vi "Vision Test.vi"() -> ()   [LabVIEW 2011]
panel:
  out "Number of Targets":i32(slide) scale=0.005..5.0
  in  "Margin of Error":i32=25
  in  "Draw Targets":bool
  out "Procesing Time":cluster{"Procesing Time":u32, "CAi":dbl}(graph)
  in  "stop":bool
  in  "Blue or Luma or Val or Inten Range":cluster{"Lower value":i32, "Upper value":i32}={"Lower value"=20, "Upper value"=120}
  in  "Green or Sat Range":cluster{"Lower value":i32, "Upper value":i32}={"Lower value"=0, "Upper value"=255}
  in  "Red or Hue Range":cluster{"Lower value":i32, "Upper value":i32}={"Lower value"=80, "Upper value"=100}
  out "ImageR":T1(plugin-control)
  out "ImageL":T1(plugin-control)
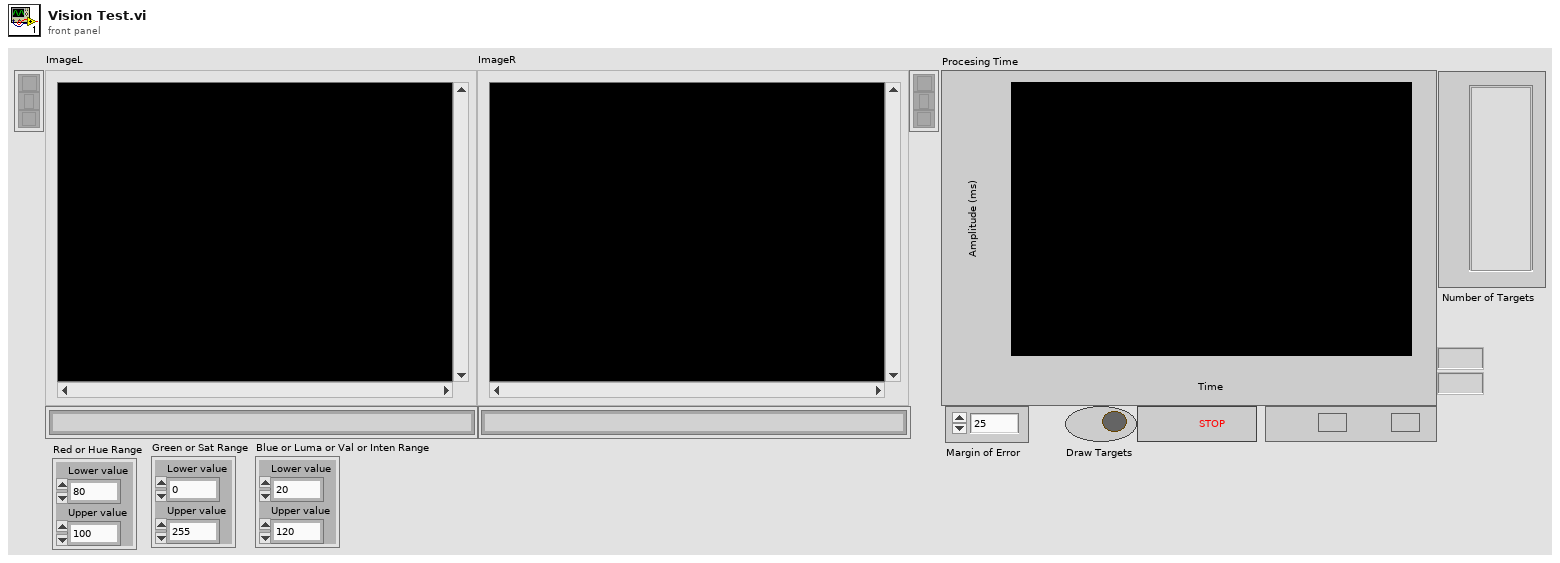
[diagram p1: front panel]
types:
  T1 = typedef "IMAQ Image.ctl" = refnum<image>
  T2 = typedef "Image Type" = u32
  T3 = cluster{"LeftImage_Mark":cluster{"Blob":cluster{"Center of Mass":cluster{"X":dbl, "Y":dbl}, "First Pixel":cluster{"X":dbl, "Y":dbl}, "Bounding Rect":cluster{"Left":dbl, "Top":dbl, "Right":dbl, "Bottom":dbl}, "Bounding Rect Size":cluster{"X":dbl, "Y":dbl}, "Area":dbl}, "Cluster":cluster{"TopLeft":cluster{"X":dbl, "Y":dbl}, "TopRight":cluster{"X":dbl, "Y":dbl}, "BottomRight":cluster{"X":dbl, "Y":dbl}, "BottomLeft":cluster{"X":dbl, "Y":dbl}}}, "RightImage_Mark":cluster{"Blob":cluster{"Center of Mass":cluster{"X":dbl, "Y":dbl}, "First Pixel":cluster{"X":dbl, "Y":dbl}, "Bounding Rect":cluster{"Left":dbl, "Top":dbl, "Right":dbl, "Bottom":dbl}, "Bounding Rect Size":cluster{"X":dbl, "Y":dbl}, "Area":dbl}, "Cluster":cluster{"TopLeft":cluster{"X":dbl, "Y":dbl}, "BottomRight":cluster{"X":dbl, "Y":dbl}, "BottomLeft":cluster{"X":dbl, "Y":dbl}, "TopRight":cluster{"X":dbl, "Y":dbl}}}, "Numeric Control":dbl}[]
  T4 = cluster{"Procesing Time":u32, "Running Average":dbl}
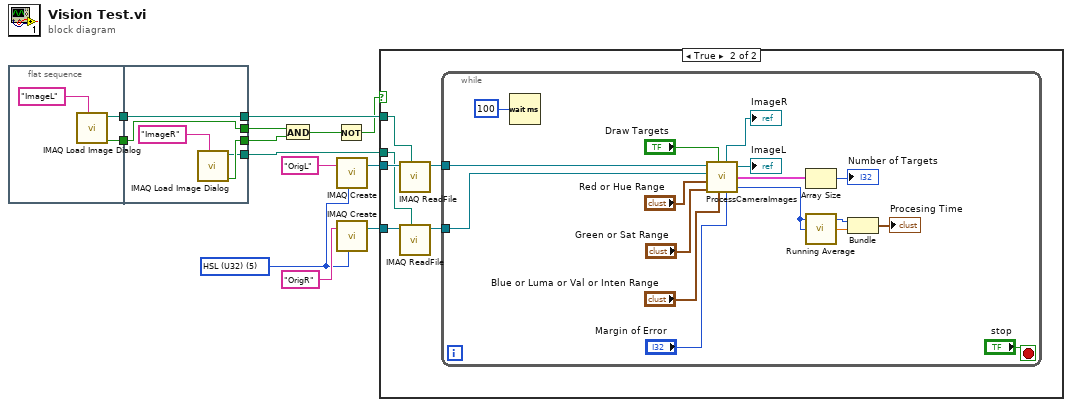
[diagram p0: block diagram]
diagram:
  w8 = T2 5 items=["Grayscale (U8)", "Grayscale (I16)", "Grayscale (SGL)", "Complex (CSG)", "RGB (U32)", "HSL (U32)", "RGB (U64)", "Grayscale (U16)"] ("Image Type")
  n1 = flat-sequence {
    tunnel: [w16] -> w4
    tunnel: [w14] -> w3
    tunnel: [w20] -> w7
    tunnel: [w21] -> w13
    tunnel: w4 -> [w21]
    tunnel: w3 -> [w20]
    tunnel: [w18] -> w2
    tunnel: [w17] -> w1
    frame #0 {
      n2 = call "IMAQ Load Image Dialog"("Prompt"="ImageL") -> ("Cancelled?"=w14:bool, "Path"=w16:path)  [unwired: 8 in, 1 out]
    }
    frame #1 {
      n3 = call "IMAQ Load Image Dialog"("Prompt"="ImageR") -> ("Cancelled?"=w18:bool, "Path"=w17:path)  [unwired: 8 in, 1 out]
    }
  }
  n4 = And(x=w7, y=w2) -> (x .and. y?=w6:bool)
  n5 = Not(x=w6) -> (.not. x?=w5:bool)
  n6 = call "IMAQ Create"("Image Name"="OrigL", "Image Type"=w8) -> ("New Image"=w12:T1)  [unwired: 3 in, 1 out]
  n7 = call "IMAQ Create"("Image Name"="OrigR", "Image Type"=w8) -> ("New Image"=w9:T1)  [unwired: 3 in, 1 out]
  n8 = case shown="True" w5 {
    tunnel: w13 -> [_ w26]
    tunnel: w12 -> [_ w27]
    tunnel: w9 -> [_ w25]
    tunnel: w1 -> [_ w24]
    frame False {
    }
    frame True {
      n9 = call "IMAQ ReadFile"("File Path"=w26, "Image"=w27) -> ("Image Out"=w23:T1)  [unwired: 5 in, 4 out]
      n10 = call "IMAQ ReadFile"("File Path"=w24, "Image"=w25) -> ("Image Out"=w22:T1)  [unwired: 5 in, 4 out]
      n11 = while {
        tunnel: w23 -> [w41]
        tunnel: w22 -> [w40]
        stop <- "stop" stop-if-true
        n12 = Wait (ms)(milliseconds to wait=u32 100) -> ()  [unwired: 1 out]
        n13 = call "ProcessCameraImages.vi"("Margin of Error"="Margin of Error", "Blue or Luma or Val or Inten Range"="Blue or Luma or Val or Inten Range", "Green or Sat Range"="Green or Sat Range", "Red or Hue Range"="Red or Hue Range", "Draw Targets"="Draw Targets", "R_Image"=w40, "L_Image"=w41) -> ("Procesing Time"=w29:u32, "TargetMatch"=w32:T3, "L_Image Out"=→"ImageL":T1, "R_Image Out"=→"ImageR":T1)
        n14 = Array Size(array=w32) -> (size(s)=→"Number of Targets":i32)
        n15 = call "Running Average.vi"("New Value"=w29) -> ("Running Average"=w28:dbl)
        n16 = Bundle("Procesing Time"=w29, "Running Average"=w28) -> (→"Procesing Time":T4)  [unwired: 1 in]
      }
    }
  }
